vi "UMB_WallAvoid.vi"(8 "tweak cluster":T1, 9 "behavior weights":i8[](array[numeric]), 10 "Boat Heading":i32, 11 "WhatAroundMeMap?":cluster{"T":dbl, "Range":dbl, "Bearing":dbl}[](array[cluster])) -> (3 "Behavior Output":T2)   [LabVIEW 2012]
uses:
  NINJA Code/Tugboat/Robo_Programs/behaviorOutput_t.ctl
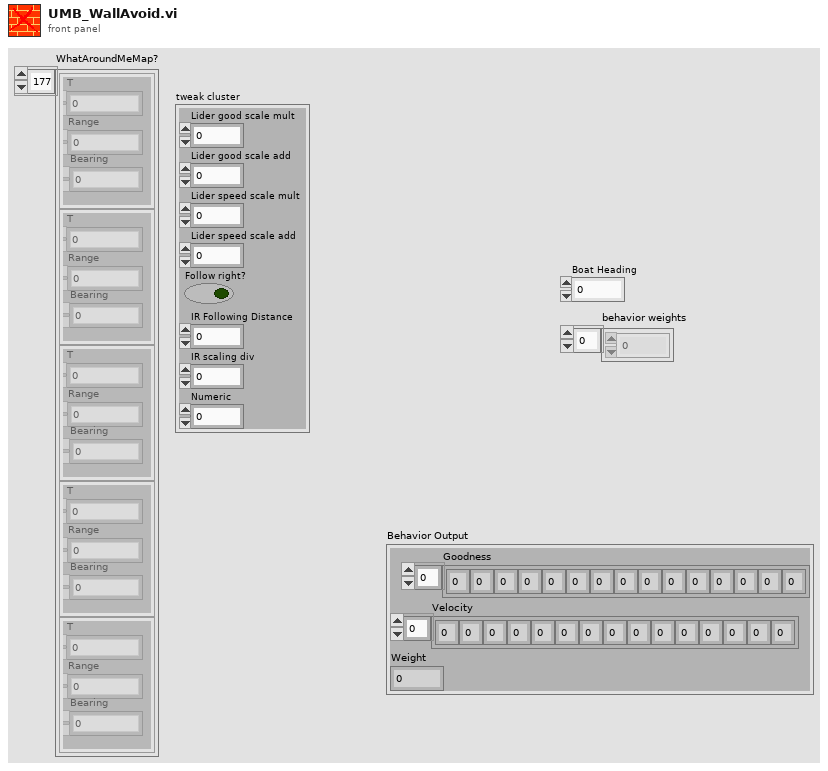
[diagram p1: front panel]
types:
  T1 = cluster{"Lider good scale mult":dbl, "Lider good scale add":dbl, "Lider speed scale mult":dbl, "Lider speed scale add":dbl, "Follow right?":bool, "IR Following Distance":i32, "IR scaling div":dbl, "Numeric":dbl}
  T2 = typedef "behaviorOutput_t.ctl" = cluster{"Goodness":i8[], "Velocity":i8[], "Weight":i8}
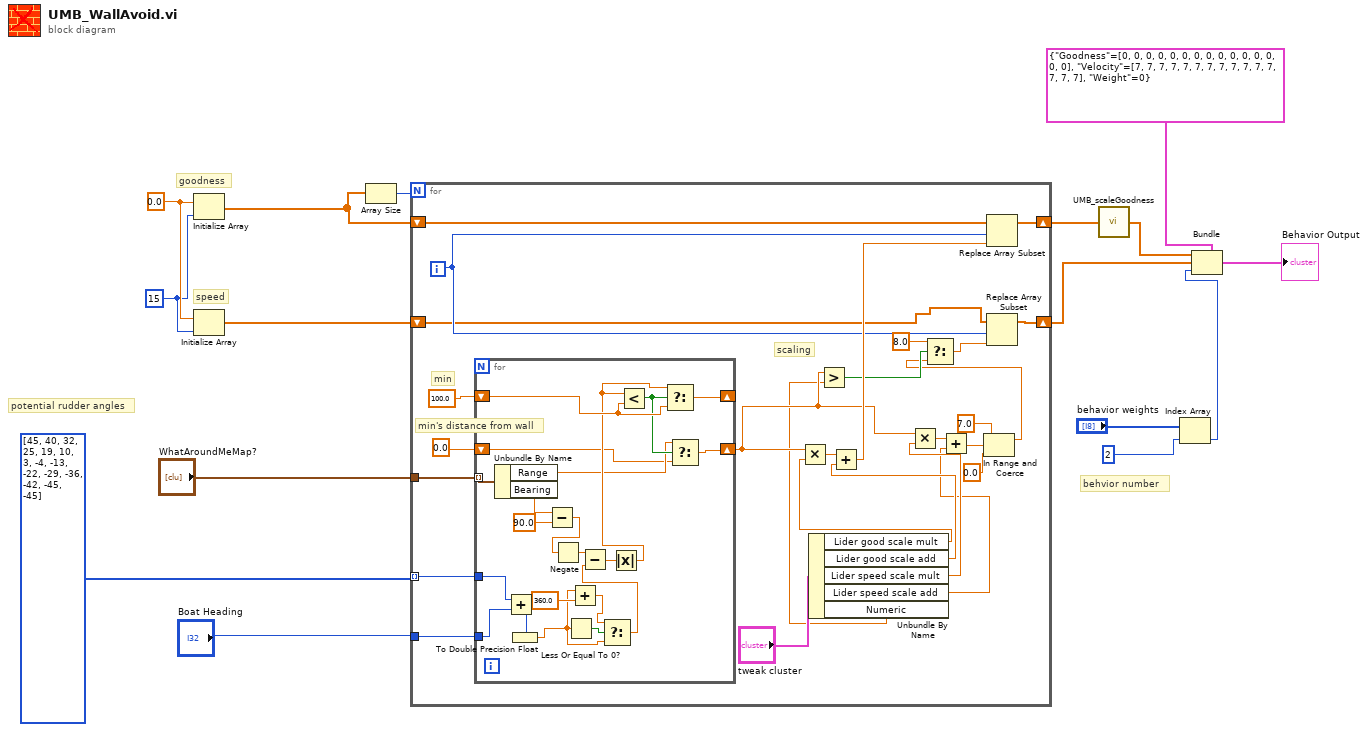
[diagram p0: block diagram]
diagram:
  w15 = 15 ("dimension size")
  w16 = 0.0 ("element")
  # "potential rudder angles"
  # "behvior number"
  # "goodness"
  # "speed"
  n1 = Initialize Array(w16, w15) -> (w14:dbl[])
  n2 = Initialize Array(w16, w15) -> (w13:dbl[])
  n3 = Array Size(array=w14) -> (size(s)=w12:i32)
  n4 = for {
    N: w12 -> [_]
    shift-right: [w42] -> w11
    shift-left: w14 -> [w43]
    shift-right: [w41] -> w7
    shift-left: w13 -> [w27]
    tunnel: i32[] [45, 40, 32, 25, 19, 10, 3, -4, -13, -22, -29, -36, -42, -45, -45] -> [w39] mode=indexing
    tunnel: "Boat Heading" -> [w40]
    tunnel: "WhatAroundMeMap?" -> [w38]
    i -> [w32]
    # "scaling"
    # "min's distance from wall"
    # "min"
    n5 = for {
      tunnel: w40 -> [w64]
      tunnel: w39 -> [w63]
      tunnel: w38 -> [w62] mode=indexing
      shift-right: [w59] -> _
      shift-left: 100.0 -> [w58]
      shift-right: [w56] -> w21
      shift-left: 0.0 -> [w53]
      n6 = Unbundle By Name(w62) -> ("Range"=w54:dbl, "Bearing"=w48:dbl)
      n7 = Add(x=w63, y=w64) -> (x+y=w61:i32)
      n8 = To Double Precision Float(number=w61) -> (double precision float=w50:dbl)
      n9 = Subtract(x=w48, y=90.0) -> (x-y=w45:dbl)
      n10 = Negate(x=w45) -> (-x=w46:dbl)
      n11 = Less Or Equal To 0?(x=w50) -> (x <= 0?=w44:bool)
      n12 = Add(x=w50, y=360.0) -> (x+y=w51:dbl)
      n13 = Select(t=w51, s=w44, f=w50) -> (s? t:f=w49:dbl)
      n14 = Subtract(x=w46, y=w49) -> (x-y=w60:dbl)
      n15 = Absolute Value(x=w60) -> (abs(x)=w57:dbl)
      n16 = Less?(x=w57, y=w58) -> (x < y?=w55:bool)
      n17 = Select(t=w57, s=w55, f=w58) -> (s? t:f=w59:dbl)
      n18 = Select(t=w54, s=w55, f=w53) -> (s? t:f=w56:dbl)
    }
    n19 = Unbundle By Name("tweak cluster") -> ("Lider good scale mult"=w31:dbl, "Lider good scale add"=w30:dbl, "Lider speed scale mult"=w29:dbl, "Lider speed scale add"=w28:dbl, "Numeric"=w17:dbl)
    n20 = Multiply(x=w21, y=w31) -> (x*y=w35:dbl)
    n21 = Greater?(x=w21, y=w17) -> (0:w20:bool)
    n22 = Add(x=w35, y=w30) -> (x+y=w34:dbl)
    n23 = Multiply(x=w21, y=w29) -> (x*y=w33:dbl)
    n24 = Add(x=w33, y=w28) -> (x+y=w26:dbl)
    n25 = In Range and Coerce(upper limit=7.0, x=w26, lower limit=0.0) -> (coerced(x)=w19:dbl)  [unwired: 1 out]
    n26 = Select(t=8.0, s=w20, f=w19) -> (s? t:f=w22:dbl)
    n27 = Replace Array Subset(array=w43, new element=w34, index=w32) -> (w42:dbl[])
    n28 = Replace Array Subset(array=w27, new element=w22, index=w32) -> (w41:dbl[])
  }
  n29 = call "UMB_scaleGoodness.vi"("goodness"=w11) -> ("scaled goodness"=w8:dbl[])
  n30 = Index Array(array="behavior weights", index=2) -> (element=w4:i8)
  n31 = Bundle(cluster=T2 {"Goodness"=[0, 0, 0, 0, 0, 0, 0, 0, 0, 0, 0, 0, 0, 0, 0], "Velocity"=[7, 7, 7, 7, 7, 7, 7, 7, 7, 7, 7, 7, 7, 7, 7], "Weight"=0} ("Behavior Output"), "Goodness"=w8, "Velocity"=w7, "Weight"=w4) -> (→"Behavior Output":T2)
